vi "Write Key DBL.vi"(7 "Section Name":string, 8 "error in":errorcluster, 9 "New Value":dbl, 10 "Key Name":string, 11 "Config File.lvclass in":T1) -> (0 "error out":errorcluster, 3 "Config File.lvclass out":T1)   [LabVIEW 2017]
uses:
  Config Cluster.ctl
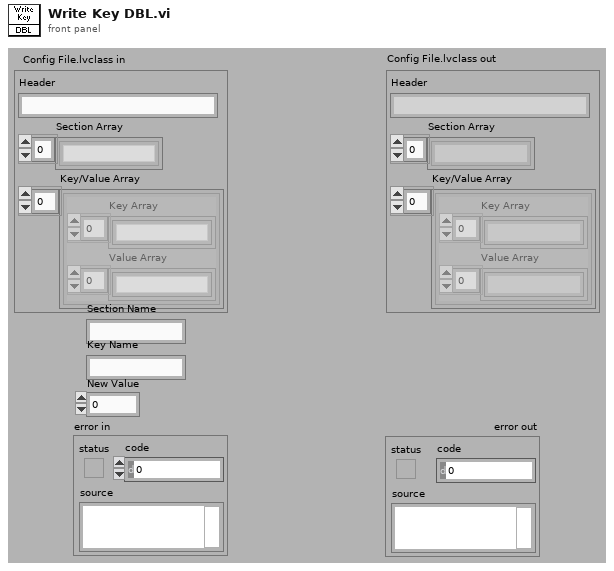
[diagram p1: front panel]
types:
  T1 = typedef "Config Cluster.ctl" = cluster{"Header":string, "Section Array":string[], "Key/Value Array":cluster{"Key Array":string[], "Value Array":string[]}[]}
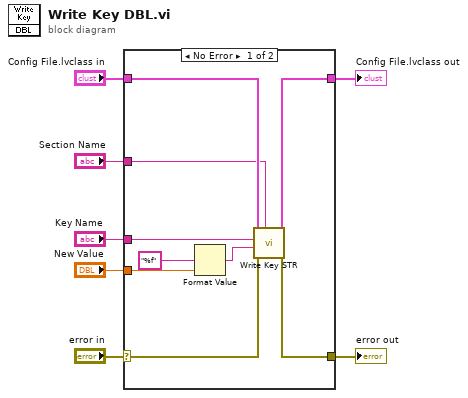
[diagram p0: block diagram]
diagram:
  n1 = case shown="No Error" "error in" {
    selector: "error in" -> [w8 w17]
    tunnel: [w9 w17] -> w6
    tunnel: "Config File.lvclass in" -> [w12 w18]
    tunnel: [w10 w18] -> w4
    tunnel: "Section Name" -> [w11 _]
    tunnel: "Key Name" -> [w13 _]
    tunnel: "New Value" -> [w15 _]
    frame No Error {
      n2 = Format Value(format string="%f", value (0)=w15) -> (output string=w14:string)  [unwired: 1 in]
      n3 = call "Write Key STR.vi"("Section Name"=w11, "error in"=w8, "New Value"=w14, "Key Name"=w13, "Config Cluster in"=w12) -> ("error out"=w9:errorcluster, "Config Cluster out"=w10:T1)  [unwired: 5 in]
    }
    frame Error {
    }
  }
  "error out" <- w6
  "Config File.lvclass out" <- w4
